vi "Save Waveform Chart history - multiple plots.vi"(8 "error in (no error)":errorcluster, 9 "History Data - multiple plots":waveform(dbl)[][](array[waveform]), 10 "Plot GUI label":string, 11 "Father of all uServices in":refnum<class "Father of all uServices.lvclass">) -> (0 "error out":errorcluster, 3 "Father of all uServices out":refnum<class "Father of all uServices.lvclass">)   [LabVIEW 2026, in "TALOS.lvlib" / "Father of all uServices.lvlib" / "Father of all uServices.lvclass"]
uses:
  Father of all uServices.lvclass
  Waveform Chart Class Reference Strict - multiple plots.ctl
  Ancestor/Ancestor/Ancestor.lvclass/Ancestor.ctl
  Support VIs/Generate Error.vi
  FGV/Error Memory/Get Error Description.vi
  Support VIs/Get PC name.vi
  Ancestor/Ancestor/Read ID.vi
  Support VIs/Get Class Name.vi
  <vilib>/Utility/error.llb/Clear Errors.vi
  FGV/Error Memory/Error Memory Core.vi
  <vilib>/AdvancedString/Delimited String to 1D String Array.vi
  <vilib>/AdvancedString/Delimited String to 1D String Array (string).vi
  Support VIs/Circus Root Path.vi
  FGV/Error Memory/Error Crt Lvl checker.vi
  FGV/Error Memory/Error Memory Core.vi/40c8088d-b597-4017-91af-faa98e00292e.vi
  FGV/Error Memory/Error Memory Core.vi/d4a3ab98-063c-4e44-b43d-fbdcfe6c2be2.vi
  <vilib>/Utility/file.llb/Write Delimited Spreadsheet (DBL).vi
  Support VIs/Global Memory.vi
  <vilib>/Utility/LVClass/Get LV Class Name.vi
  Support VIs/Is in Packed Library.vi
  Support VIs/TALOS Root path.vi
  Support VIs/Read CSV worksheet.vi
  Support VIs/Global Constants.vi
  <vilib>/Utility/error.llb/General Error Handler.vi
  Support VIs/Error Log.vi
  Ancestor/Ancestor/Ancestor.lvclass
  <vilib>/Comparison/Equal/Equal Functor/Equal Functor.lvclass
  TALOS.lvlib
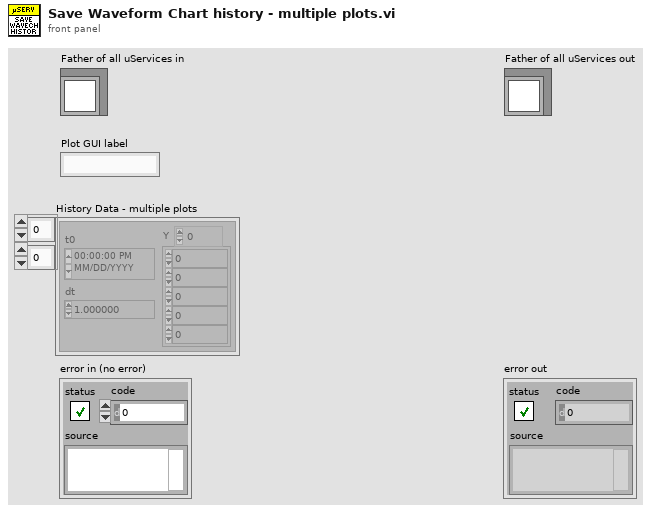
[diagram p1: front panel]
types:
  T1 = typedef "TALOS.lvlib/Father of all uServices.lvlib/Father of all uServices.lvclass/Waveform Chart Class Reference Strict - multiple plots.ctl" = refnum<vi>
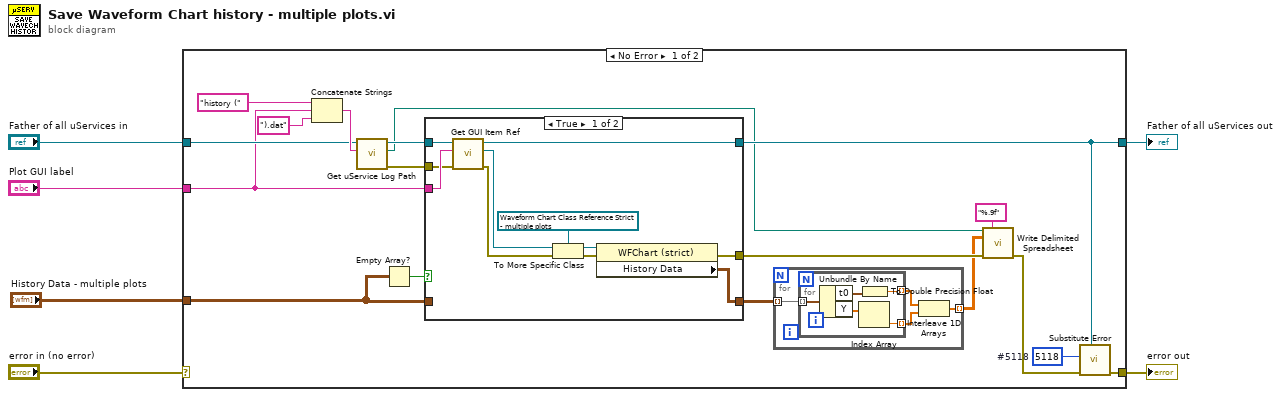
[diagram p0: block diagram]
diagram:
  n1 = case shown="No Error" "error in (no error)" {
    selector: "error in (no error)" -> [_ w49]
    tunnel: [w20 w49] -> w5
    tunnel: [w14 w48] -> w3
    tunnel: "Father of all uServices in" -> [w17 w48]
    tunnel: "Plot GUI label" -> [w13 _]
    tunnel: "History Data - multiple plots" -> [w15 _]
    frame No Error {
      w19 = 5118  # #5118
      n2 = Concatenate Strings("history (" ("string"), w13, ").dat" ("string")) -> (w21:string)
      n3 = call "Get uService Log Path.vi"("Log File Suffix"=w21, "Father of all uServices in"=w17) -> ("error out"=w12:errorcluster, "Log File Path"=w9:path, "Father of all uServices out"=w16:refnum<class "Father of all uServices.lvclass">)  [unwired: 7 in]
      n4 = Empty Array?(array=w15) -> (empty?=w18:bool)
      n5 = case shown="True" w18 {
        tunnel: [w44 w45] -> w24
        tunnel: w16 -> [w40 w46]
        tunnel: w15 -> [_ w47]
        tunnel: [w39 w46] -> w14
        tunnel: w13 -> [w38 _]
        tunnel: [w36 w47] -> w11
        tunnel: w12 -> [w35 w45]
        frame True {
          n6 = call "Get GUI Item Ref.vi"("error in (no error)"=w35, "FP Item Name"=w38, "uService Template in"=w40) -> ("error out"=w34:errorcluster, "Ctl Refnum"=w37:refnum<vi>, "uService Template out"=w39:refnum<class "Father of all uServices.lvclass">)  [unwired: 6 in]
          n7 = To More Specific Class(target class=T1 refnum ("Waveform Chart - multiplot"), reference=w37, error in=w34) -> (specific class reference=w43:T1, error out=w42:errorcluster)
          n8 = property class="WFChart (strict)"(reference=w43, error in=w42) -> (error out=w44:errorcluster, "History Data"=w36:waveform(dbl)[][])  [unwired: 1 out]
        }
        frame False {
        }
      }
      n9 = for {
        tunnel: w11 -> [w28] mode=indexing
        tunnel: [w25] -> w10 mode=indexing
        n10 = for {
          tunnel: w28 -> [w33] mode=indexing
          tunnel: [w30] -> w27 mode=indexing
          tunnel: [w29] -> w26 mode=indexing
          n11 = Unbundle By Name(w33) -> ("t0"=w31:timestamp, "Y"=w32:dbl[])
          n12 = Index Array(array=w32) -> (element=w29:dbl)  [unwired: 1 in]
          n13 = To Double Precision Float(number=w31) -> (double precision float=w30:dbl)
        }
        n14 = Interleave 1D Arrays(w27, w26) -> (w25:dbl[])
      }
      n15 = call-poly <vilib>:"Write Delimited Spreadsheet.vi"("file path (dialog if empty)"=w9, "format (%.3f)"="%.9f", "2D data"=w10, "error in (no error)"=w24) -> ("error out"=w8:errorcluster)  [unwired: 10 in, 1 out]
      n16 = call "Substitute Error.vi"("LabVIEW Object"=w14, "error in (no error)"=w8, "Error Code"=w19) -> ("error out"=w20:errorcluster)  [unwired: 8 in]
    }
    frame Error {
    }
  }
  "error out" <- w5
  "Father of all uServices out" <- w3
